vi "Law of Cosines.vi"(1 "c":dbl, 2 "b":dbl, 3 "a":dbl) -> (0 "Gamma":dbl)   [LabVIEW 2011]
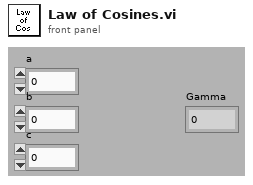
[diagram p1: front panel]
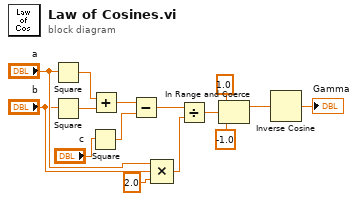
[diagram p0: block diagram]
diagram:
  n1 = Square(x="a") -> (x^2=w9:dbl)
  n2 = Square(x="b") -> (x^2=w8:dbl)
  n3 = Square(x="c") -> (x^2=w5:dbl)
  n4 = Add(x=w9, y=w8) -> (x+y=w12:dbl)
  n5 = Subtract(x=w12, y=w5) -> (x-y=w13:dbl)
  n6 = Compound Arithmetic op=MULTIPLY("a", "b", 2.0 ("value")) -> (w14:dbl)
  n7 = Divide(x=w13, y=w14) -> (x/y=w4:dbl)
  n8 = In Range and Coerce(upper limit=1.0, x=w4, lower limit=-1.0) -> (coerced(x)=w3:dbl)  [unwired: 1 out]
  n9 = Inverse Cosine(1:w3) -> (0:→"Gamma":dbl)
